vi "Tester Events - Create.vi"(8 "error in":errorcluster) -> (0 "error out":errorcluster)   [LabVIEW 2024, in "Tester InterComm.lvlib"]
uses:
  Tester InterComm.lvlib
  General Actions.ctl
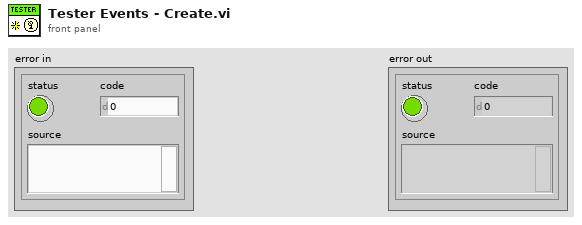
[diagram p1: front panel]
types:
  T1 = typedef "Tester InterComm.lvlib/General Actions.ctl" = enum16{"Create", "Get", "Destroy"}
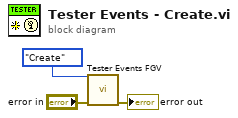
[diagram p0: block diagram]
diagram:
  n1 = call "Tester Events FGV.vi"("error in"="error in", "Action"=General_Actions."Create") -> ("error out"=→"error out":errorcluster)  [unwired: 8 in, 1 out]
